vi "Case.vi"() -> ()   [LabVIEW 2023]
panel:
  in  "Numeric":i32
  out "C 2":dbl
  in  "B 2":dbl
  in  "A 2":dbl
  out "C":dbl
  in  "Boolean":bool
  in  "B":dbl
  in  "A":dbl
  # "0(기본) : 더하기\n\n1 : 빼기\n\n11 : 곱하기\n\n-11 : 나누기"
  # "참 : 더하기\n\n거짓 : 빼기"
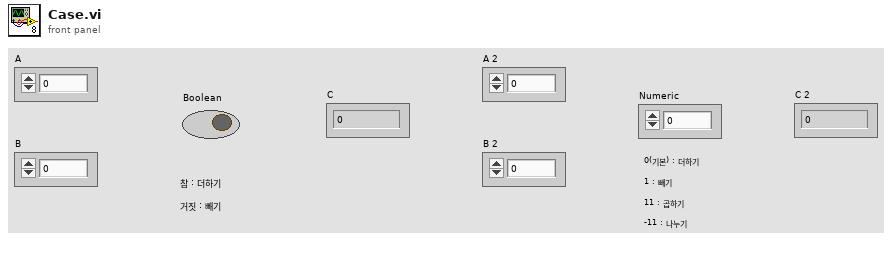
[diagram p1: front panel]
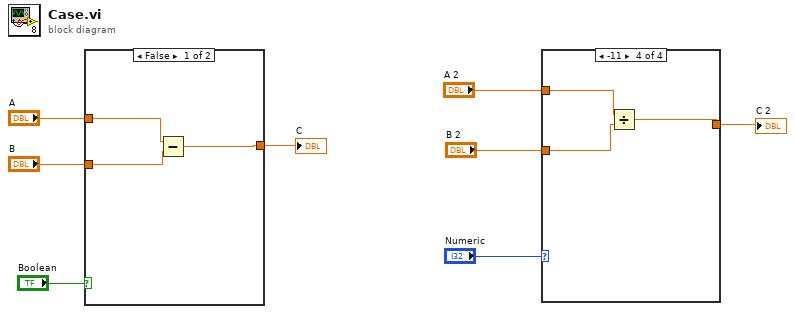
[diagram p0: block diagram]
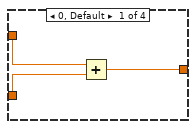
[diagram p2: hidden frame]
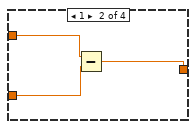
[diagram p3: hidden frame]
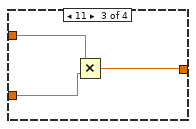
[diagram p4: hidden frame]
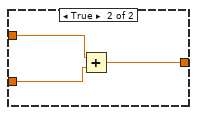
[diagram p5: hidden frame]
diagram:
  n1 = case shown="False" "Boolean" {
    tunnel: "A" -> [w11 w14]
    tunnel: "B" -> [w10 w13]
    tunnel: [w9 w12] -> w5
    frame False {
      n2 = Subtract(x=w11, y=w10) -> (x-y=w9:dbl)
    }
    frame True {
      n3 = Add(x=w14, y=w13) -> (x+y=w12:dbl)
    }
  }
  "C" <- w5
  n4 = case shown="-11" "Numeric" {
    tunnel: "A 2" -> [w17 w20 w22 w26]
    tunnel: "B 2" -> [w16 w19 w23 w25]
    tunnel: [w15 w18 w21 w24] -> w1
    frame 0, Default {
      n5 = Add(x=w17, y=w16) -> (x+y=w15:dbl)
    }
    frame 1 {
      n6 = Subtract(x=w20, y=w19) -> (x-y=w18:dbl)
    }
    frame 11 {
      n7 = Multiply(x=w22, y=w23) -> (x*y=w21:dbl)
    }
    frame -11 {
      n8 = Divide(x=w26, y=w25) -> (x/y=w24:dbl)
    }
  }
  "C 2" <- w1
